vi "ATF-Pump-Abort Executer.vi"(8 "error in":errorcluster) -> (0 "error IO":errorcluster)   [LabVIEW 2022 SP3]
uses:
  <vilib>/Platform/TimedLoop/XDataNode/timing_clust.ctl
  <vilib>/Platform/TimedLoop/XDataNode/nitl_modes.ctl
  <vilib>/Platform/TimedLoop/XDataNode/wakeup.ctl
  <vilib>/platform/TimedLoop/XDataNode/XDataNode.xnode
  <vilib>/Platform/TimedLoop/XDataNode/XDNodeRunTimeDep.lvlib
panel:
  out "Numeric":i32
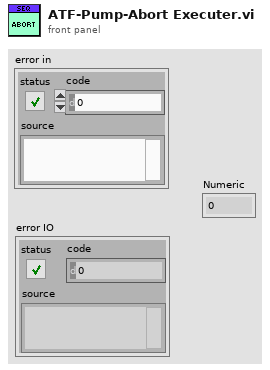
[diagram p1: front panel]
types:
  T1 = typedef "XDNodeRunTimeDep.lvlib/timing_clust.ctl" = cluster{"Expected End [f-1]":u64, "Actual End [f-1]":u64, "Finished Late? [f-1]":bool, "Expected End [i-1]":u64, "Actual End [i-1]":u64, "Finished Late? [i-1]":bool, "Expected Start [i]":u64, "Actual Start [i]":u64, "Expected Start [f]":u64, "Actual Start [f]":u64, "Source Name":string, "Structure Name":string, "Period":i64, "Deadline":i64, "Offset":i64, "Start":i64, "Priority":i32, "Timeout":i32, "Mode":T2, "Wakeup Reason":T3, "Error":errorcluster, "Source Type":string, "Secondary Source Type":string, "Global End Time":u64, "Global Start Time":u64, "Frame Duration":u64, "Iteration Duration":u64, "Assigned CPU":i32, "I/O Scan Engine Mode":u32}
  T2 = typedef "XDNodeRunTimeDep.lvlib/nitl_modes.ctl" = enum32{"No Change", "Process missed periods, maintain original phase", "Discard missed periods, maintain original phase", "Process missed periods, ignore original phase", "Discard missed periods, ignore original phase"}
  T3 = typedef "XDNodeRunTimeDep.lvlib/wakeup.ctl" = enum32{"Normal", "Aborted", "Asynchronous wakeup", "Timing source error", "Timed loop error", "Timeout"}
  T4 = enum16{"Init", "Read", "Write 'All'", "Write 'n'", "Write Safe Value", "Write Start Time", "Overwrite Pattern", "Overwrite Pattern with Start", "Append Pattern", "Start Pattern Mode", "Abort Pattern Mode", "Read 1"}
  T5 = cluster{"Start DAQ":bool, "Stop DAQ":bool, "RT Stop":bool, "RT Exit":bool, "Start Seq":bool}
  T6 = cluster{"Manual HOLD":bool, "Automatic Hold AI":bool, "Abort":bool, "Automatic Hold DI":bool}
  T7 = cluster{cluster{"Sr. No.":string, "Time CDT":string, "Component ID":string, "Data Type":string, "Condition":string, "Range/Position":string, "No of Samples for Pass":string, "Event Duration":string, "Continuous /Cumulative":string, "Expected Delay":string, "Failure case Seq":string, "Current Sequence":string}[]}[]
  T8 = cluster{"Sr. No.":string, "Time CDT":string, "Component ID":string, "Data Type":string, "Condition":string, "Range/Position":string, "No of Samples for Pass":string, "Event Duration":string, "Continuous /Cumulative":string, "Expected Delay":string, "Failure case Seq":string, "Current Sequence":string}[]
  T9 = cluster{"Sr. No.":string, "Time CDT":string, "Component ID":string, "Data Type":string, "Condition":string, "Range/Position":string, "No of Samples for Pass":string, "Event Duration":string, "Continuous /Cumulative":string, "Expected Delay":string, "Failure case Seq":string, "Current Sequence":string}
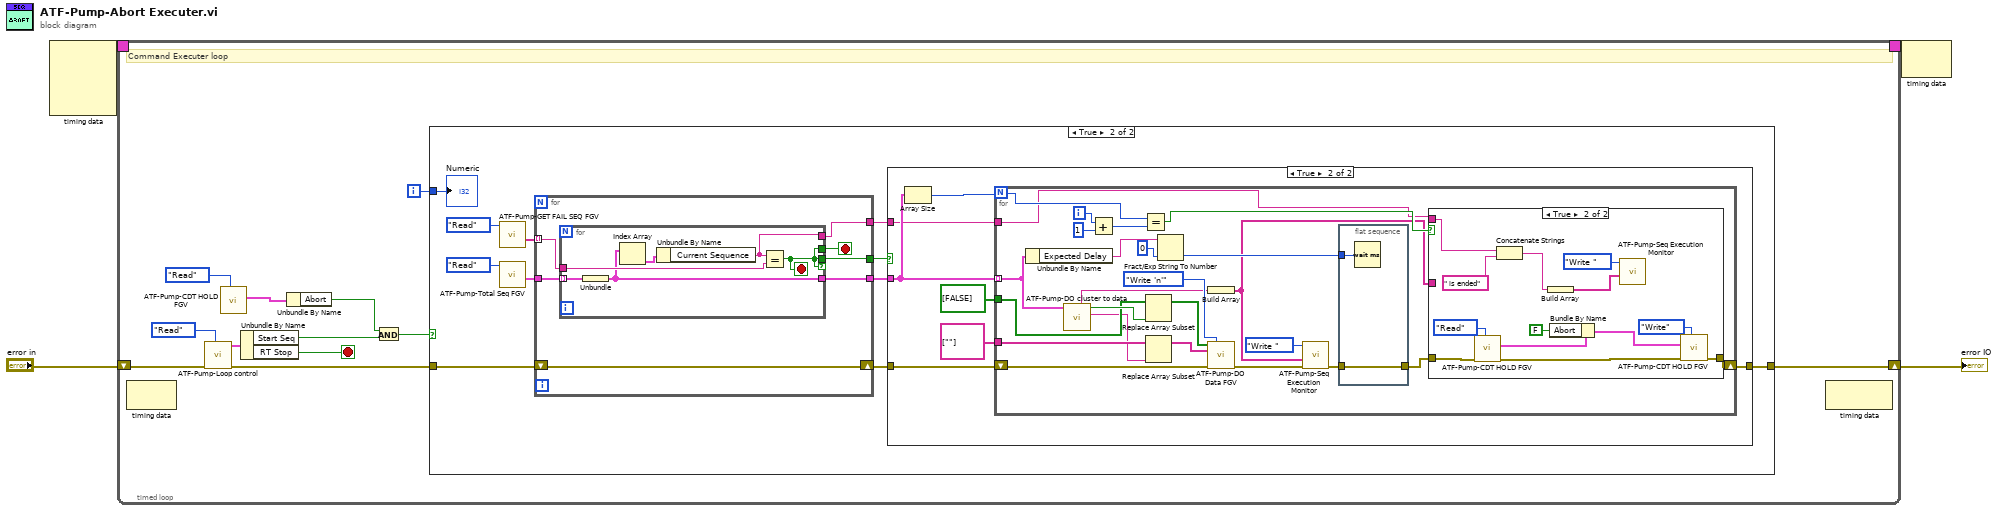
[diagram p0: block diagram]
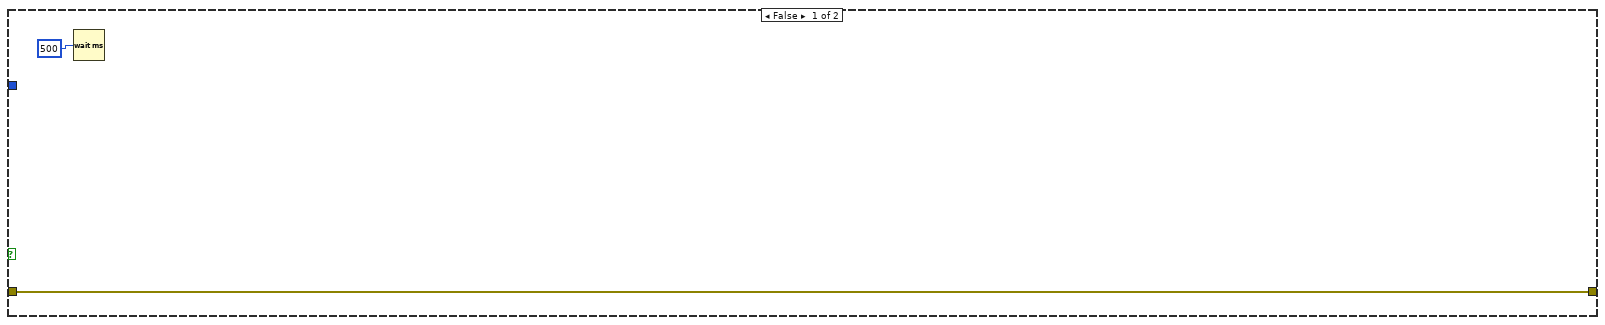
[diagram p2: hidden frame]
diagram:
  n1 = node-c288() -> (w2:T1)  [unwired: 4 in]
  n2 = timed-loop {
    shift-right: [w10] -> w3
    shift-left: "error in" -> [w14]
    timing: w2 -> [_]
    timing-out: [_] -> w1
    i -> [w15]
    stop <- w16 stop-if-true
    # "Command Executer loop"
    n3 = node-c288() -> ()  [unwired: 1 in, 1 out]
    n4 = call "ATF-Pump-Loop control.vi"("Action"=enum16{"Init", "Write", "Read"}."Read", "error in (no error)"=w14) -> ("error Out"=w13:errorcluster, "Loop Control out"=w11:T5)  [unwired: 8 in]
    n5 = call "ATF-Pump-CDT HOLD FGV.vi"("Write/Read"=enum16{"Write", "Read"}."Read") -> ("HOLD and Abort Out"=w7:T6)  [unwired: 7 in, 1 out]
    n6 = Unbundle By Name(w11) -> ("Start Seq"=w8:bool, "RT Stop"=w16:bool)
    n7 = Unbundle By Name(w7) -> ("Abort"=w5:bool)
    n8 = And(x=w5, y=w8) -> (x .and. y?=w6:bool)
    n9 = case shown="True" w6 {
      tunnel: [w18 w29] -> w10
      tunnel: w15 -> [_ w28]
      tunnel: w13 -> [w18 w21]
      frame False {
        n10 = Wait (ms)(milliseconds to wait=u32 500) -> ()  [unwired: 1 out]
      }
      frame True {
        n11 = call "ATF-Pump-GET FAIL SEQ FGV.vi"("Enum"=enum16{"Read", "Write "}."Read") -> ("Failure \ncase Seq"=w22:string[])  [unwired: 9 in, 1 out]
        n12 = call "ATF-Pump-Total Seq FGV.vi"("Enum"=enum16{"Read", "Write "}."Read") -> ("Total Seq  Out"=w25:T7)  [unwired: 9 in, 1 out]
        n13 = for {
          tunnel: [w32] -> w23
          tunnel: w25 -> [w33]
          tunnel: w22 -> [w36] mode=indexing
          tunnel: [w35] -> w24
          shift-right: [w31] -> w20
          shift-left: w21 -> [w31]
          tunnel: [w30] -> w19
          stop <- w34 stop-if-true
          n14 = for {
            tunnel: [w41] -> w35 if=w41
            tunnel: w36 -> [w42]
            tunnel: [w41] -> w34
            tunnel: w33 -> [w39] mode=indexing
            tunnel: [w38] -> w32
            tunnel: [w37] -> w30
            stop <- w41 stop-if-true
            n15 = Unbundle(w39) -> (w38:T8)
            n16 = Index Array(array=w38) -> (element=w40:T9)  [unwired: 1 in]
            n17 = Unbundle By Name(w40) -> ("Current Sequence"=w37:string)
            n18 = Equal?(x=w37, y=w42) -> (x = y?=w41:bool)
          }
        }
        n19 = case shown="True" w24 {
          tunnel: w20 -> [w43 w47]
          tunnel: [w43 w50] -> w29
          tunnel: w23 -> [_ w46]
          tunnel: w19 -> [_ w44]
          frame False {
          }
          frame True {
            n20 = Array Size(array=w46) -> (size(s)=w45:i32)
            n21 = for {
              N: w45 -> [w56]
              tunnel: w46 -> [w67] mode=indexing
              tunnel: string[] [""] ("appended array") -> [w75]
              tunnel: bool[] [FALSE] ("appended array") -> [w73]
              shift-right: [w53] -> w50
              shift-left: w47 -> [w68]
              tunnel: w44 -> [w52]
              i -> [w59]
              n22 = Unbundle By Name(w67) -> ("Expected Delay"=w70:string)
              n23 = call "ATF-Pump-DO cluster to data.vi"("output cluster"=w67) -> ("Component ID"=w63:string, "Boolean"=w74:bool, "Sequence"=w60:string)  [unwired: 7 in, 1 out]
              n24 = Add(x=w59, y=1) -> (x+y=w57:i32)
              n25 = Equal?(x=w56, y=w57) -> (x = y?=w55:bool)
              n26 = Replace Array Subset(array=w73, new element=w74) -> (w72:bool[])  [unwired: 1 in]
              n27 = Replace Array Subset(array=w75, new element=w63) -> (w71:string[])  [unwired: 1 in]
              n28 = Fract/Exp String To Number(string=w70, default (0 dbl)=u32 0 ("y")) -> (number=w65:u32)  [unwired: 2 in, 1 out]
              n29 = Build Array(w60) -> (w51:string[])
              n30 = call "ATF-Pump-DO Data FGV.vi"("DO Values In"=w72, "Option"=T4."Write 'n'", "DO Channel Names"=w71, "error in (no error)"=w68) -> ("error out"=w62:errorcluster)  [unwired: 5 in, 6 out]
              n31 = call "ATF-Pump-Seq Execution Monitor.vi"("error in"=w62, "Seq Monitor"=w51, "Enum"=enum16{"Read", "Write "}."Write ") -> ("error out"=w61:errorcluster)  [unwired: 7 in, 1 out]
              n32 = flat-sequence {
                tunnel: w61 -> [w91]
                tunnel: [w91] -> w54
                tunnel: w65 -> [w90]
                frame #0 {
                  n33 = Wait (ms)(milliseconds to wait=w90) -> ()  [unwired: 1 out]
                }
              }
              n34 = case shown="True" w55 {
                tunnel: w54 -> [w76 w86]
                tunnel: [w76 w88] -> w53
                tunnel: w52 -> [_ w80]
                tunnel: w51 -> [_ _]
                frame False {
                }
                frame True {
                  n35 = call "ATF-Pump-CDT HOLD FGV.vi"("Write/Read"=enum16{"Write", "Read"}."Read", "error in (no error)"=w86) -> ("error Out"=w85:errorcluster, "HOLD and Abort Out"=w84:T6)  [unwired: 6 in]
                  n36 = Concatenate Strings(w80, " is ended" ("string")) -> (w78:string)
                  n37 = Build Array(w78) -> (w77:string[])
                  n38 = Bundle By Name(cluster=w84, "Abort"=FALSE) -> (w82:T6)
                  n39 = call "ATF-Pump-Seq Execution Monitor.vi"("Seq Monitor"=w77, "Enum"=enum16{"Read", "Write "}."Write ") -> ()  [unwired: 8 in, 2 out]
                  n40 = call "ATF-Pump-CDT HOLD FGV.vi"("Write/Read"=enum16{"Write", "Read"}."Write", "error in (no error)"=w85, "HOLD and Abort"=w82) -> ("error Out"=w88:errorcluster)  [unwired: 5 in, 1 out]
                }
              }
            }
          }
        }
        "Numeric" <- w28
      }
    }
    n41 = node-c288() -> ()  [unwired: 1 in, 1 out]
  }
  "error IO" <- w3
  n42 = node-c288(w1) -> ()  [unwired: 1 out]
